vi "visualyze_audio_data.vi"(8 "error in (no error)":errorcluster, 10 "audio data":waveform(dbl)[](array[waveform]), 11 "Button refs In":T1) -> (0 "error out":errorcluster)   [LabVIEW 2020]
uses:
  CTLs/ButtonRefs.ctl
  CTLs/playback status.ctl
  FGVs/FGVstates.ctl
  <vilib>/Analysis/2dsp.llb/Real FFT.vi
  <vilib>/Analysis/NI_AALPro.lvlib
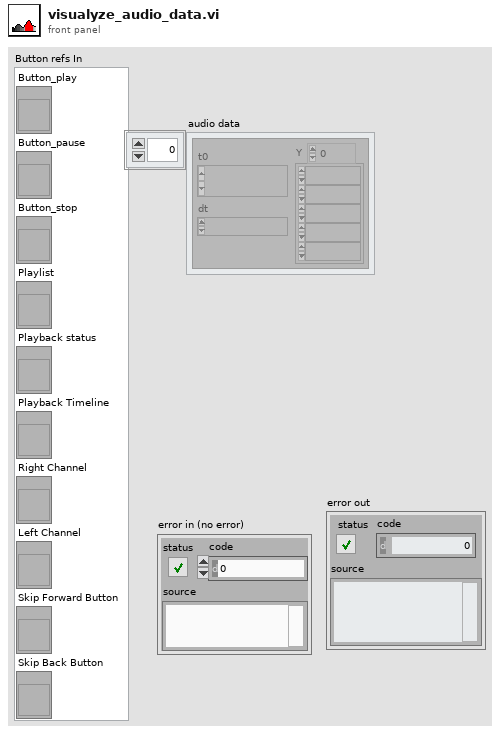
[diagram p1: front panel]
types:
  T1 = typedef "ButtonRefs.ctl" = cluster{"Button_play":refnum<vi>, "Button_pause":refnum<vi>, "Button_stop":refnum<vi>, "Playlist":refnum<vi>, "Playback status":refnum<vi>, "Playback Timeline":refnum<vi>, "Right Channel":refnum<vi>, "Left Channel":refnum<vi>, "Skip Forward Button":refnum<vi>, "Skip Back Button":refnum<vi>}
  T2 = typedef "FGVstates.ctl" = enum16{"Init", "Set", "Get", "De-Init"}
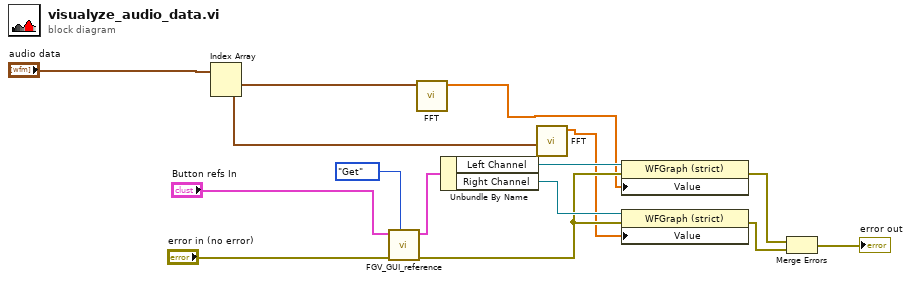
[diagram p0: block diagram]
diagram:
  n1 = Index Array(array="audio data") -> (element #1=w4:waveform(dbl), element #2=w2:waveform(dbl))  [unwired: 2 in]
  n2 = call "FGV_GUI_reference.vi"("FGV states"=FGVstates."Get", "error in (no error)"="error in (no error)", "Button refs In"="Button refs In") -> ("error out"=w9:errorcluster, "Button refs Out"=w13:T1)  [unwired: 7 in]
  n3 = call-poly <vilib>:"FFT.vi"("X"=w4) -> ("FFT {X}"=w3:cdb[])  [unwired: 9 in, 1 out]
  n4 = Unbundle By Name(w13) -> ("Left Channel"=w12:refnum<vi>, "Right Channel"=w11:refnum<vi>)
  n5 = call-poly <vilib>:"FFT.vi"("X"=w2) -> ("FFT {X}"=w1:cdb[])  [unwired: 9 in, 1 out]
  n6 = property class="WFGraph (strict)"(reference=w12, error in=w9, "Value"=w3) -> (error out=w8:errorcluster)  [unwired: 1 out]
  n7 = property class="WFGraph (strict)"(reference=w11, error in=w9, "Value"=w1) -> (error out=w6:errorcluster)  [unwired: 1 out]
  n8 = Merge Errors(w8, w6) -> (→"error out":errorcluster)
